vi "DriveModuleControl_TravTuneKsKv.vi"(8 "error in":errorcluster, 9 "Actual State":T1={"Speed"=0.0, "Angle"={"VALUE"=0.0, "COS"=1.0, "SIN"=0.0}} {"Angle"."SIN" format="%13.4f"; "Angle"."COS" format="%13.4f"; "Angle"."VALUE" format="%13.4f"}, 10 "Desired State":T1={"Speed"=0.0, "Angle"={"VALUE"=0.0, "COS"=1.0, "SIN"=0.0}} {"Angle"."SIN" format="%13.4f"; "Angle"."COS" format="%13.4f"; "Angle"."VALUE" format="%13.4f"}, 11 "ModualNamePrefix":i32) -> (0 "error out":errorcluster)   [LabVIEW 2023]
uses:
  <vilib>/Rock Robotics/WPI/ThirdParty/JAS_Junk/TrajLib/TypeDef/SWERVE_DRIVE_MODULE_STATE.ctl
  <vilib>/Rock Robotics/WPI/ThirdParty/JAS_Junk/TrajLib/TypeDef/ROTATION2D.ctl
  <vilib>/Rock Robotics/WPI/ThirdParty/JAS_Junk/TrajLib/Rotation2d_Minus.vi
  <vilib>/Rock Robotics/WPI/ThirdParty/JAS_Junk/TrajLib/Rotation2d_GetRadians.vi
  <vilib>/Rock Robotics/WPI/ThirdParty/JAS_Junk/TrajLib/SwerveModuleState_New.vi
  <vilib>/Rock Robotics/WPI/ThirdParty/JAS_Junk/TrajLib/Rotation2d_RotateBy.vi
  <vilib>/Rock Robotics/WPI/ThirdParty/JAS_Junk/TrajLib/Rotation2d_CreateAngle.vi
  <vilib>/Rock Robotics/WPI/ThirdParty/JAS_Junk/TrajLib/SimpleMotorFF_Calculate.vi
  <vilib>/Rock Robotics/WPI/ThirdParty/JAS_Junk/TrajLib/PIDController_AtSetpoint.vi
  <vilib>/Rock Robotics/WPI/ThirdParty/JAS_Junk/TrajLib/PIDController_SetPIDF.vi
  <vilib>/Rock Robotics/WPI/ThirdParty/JAS_Junk/TrajLib/PIDController_SetDerivativeFilter.vi
  <vilib>/Rock Robotics/WPI/ThirdParty/JAS_Junk/TrajLib/PIDController_SetIntegratorRange.vi
  <vilib>/Rock Robotics/WPI/ThirdParty/JAS_Junk/TrajLib/PIDController_SetTolerancePandV.vi
  <vilib>/Rock Robotics/WPI/ThirdParty/JAS_Junk/TrajLib/PIDController_DisableContinousInput.vi
  <vilib>/Rock Robotics/WPI/ThirdParty/JAS_Junk/TrajLib/PIDController_EnableContinousInput.vi
  <vilib>/Rock Robotics/WPI/ThirdParty/JAS_Junk/TrajLib/PIDController_Reset.vi
  <vilib>/Rock Robotics/WPI/ThirdParty/JAS_Junk/TrajLib/PIDController_New.vi
  <vilib>/Rock Robotics/WPI/ThirdParty/JAS_Junk/TrajLib/PIDController_SetOutputLimits.vi
  <vilib>/Rock Robotics/WPI/ThirdParty/JAS_Junk/TrajLib/VI/PIDController_SetIntegratorZone.vi
  <vilib>/Rock Robotics/WPI/ThirdParty/JAS_Junk/TrajLib/LinearFilter_ResetToValue.vi
  <vilib>/Rock Robotics/WPI/ThirdParty/JAS_Junk/TrajLib/LinearFilter_Calculate.vi
  <vilib>/Rock Robotics/WPI/ThirdParty/JAS_Junk/TrajLib/Rotation2d_UnaryMinus.vi
  <vilib>/Rock Robotics/WPI/ThirdParty/JAS_Junk/TrajLib/Rotation2d_CreateXY.vi
  <vilib>/Rock Robotics/WPI/ThirdParty/JAS_Junk/TrajLib/PIDController_NewPeriod.vi
  <vilib>/Rock Robotics/WPI/ThirdParty/JAS_Junk/TrajLib/Util_CalcDist.vi
  <vilib>/Rock Robotics/SystemInterfaces/NetworkCommunication/NetComm_UsageReport_report.vi
  DriveGlobal.vi
  <vilib>/Rock Robotics/WPI/ThirdParty/Phoenix-LabVIEW/CANCoder/CTRE_Phoenix_CANcoder_RefNumRegistryGet.vi
  <vilib>/Rock Robotics/WPI/MotorControl/WPI_MotorControlRefNum Registry Get.vi
  <vilib>/Rock Robotics/Network Tables/NT Write Number.vi
  <vilib>/Rock Robotics/WPI/ThirdParty/JAS_Junk/TrajLib/LinearFilter_MovingAverage.vi
  <vilib>/Rock Robotics/WPI/ThirdParty/JAS_Junk/TrajLib/LinearFilter_LowPassBW1.vi
  <vilib>/Rock Robotics/WPI/ThirdParty/JAS_Junk/TrajLib/LinearFilter_LowPassBW2.vi
  <vilib>/Rock Robotics/WPI/ThirdParty/JAS_Junk/TrajLib/LinearFilter_HighPassBW1.vi
  <vilib>/Rock Robotics/WPI/ThirdParty/JAS_Junk/TrajLib/LinearFilter_HighPassBW2.vi
  <vilib>/Utility/semaphor.llb/Obtain Semaphore Reference.vi
  <vilib>/Rock Robotics/WPI/ThirdParty/JAS_Junk/TrajLib/Timer_Reset.vi
  <vilib>/Rock Robotics/WPI/ThirdParty/JAS_Junk/TrajLib/Globals/Util_LibraryGlobals.vi
  <vilib>/Rock Robotics/WPI/ThirdParty/JAS_Junk/TrajLib/PIDController_AdvCalculate_FF_Sp_Pv.vi
  <vilib>/Rock Robotics/WPI/ThirdParty/JAS_Junk/TrajLib/Trajectory_Library.lvlib
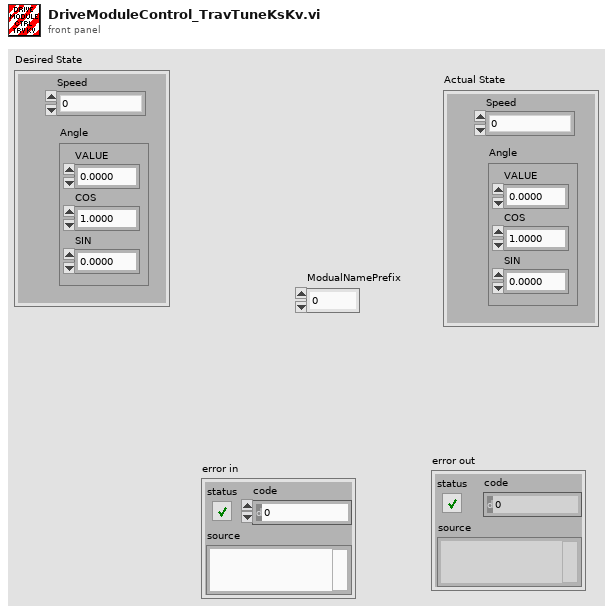
[diagram p1: front panel]
types:
  T1 = typedef "Trajectory_Library.lvlib/SWERVE_DRIVE_MODULE_STATE.ctl" = cluster{"Speed":dbl, "Angle":T2}
  T2 = typedef "Trajectory_Library.lvlib/ROTATION2D.ctl" = cluster{"VALUE":dbl, "COS":dbl, "SIN":dbl}
  T3 = enum16{"Moving Average", "Low Pass 1st Order Butterworth", "Low Pass 2nd Order Butterworth", "High Pass 1st Order Butterworth", "High Pass 2nd Order Butterworth"}
  T4 = typedef "WPI_MotorControlDeviceRef.ctl" = cluster{"DeviceStatus":errorcluster, "Type":T5, "PWM":cluster{"PWM Channel":T6, "DeadBand":T7}, "CAN":cluster{"Device Number":u8, "SetOutput VI Ref":variant, "GetOutput VI Ref":variant, "Enable VI Ref":variant, "Disable VI Ref":variant, "Data":variant}, "Invert":bool, "DIO PWM":cluster{"PWM \"Enable\" Channel":T6, "DIOChannel":T8, "PWM Rate":dbl}}
  T5 = typedef "WPI_MotorControlType.ctl" = enum16{"PWM", "CAN", "DIO PWM"}
  T6 = typedef "FPGA_DIOPWMChannel.ctl" = enum8{"PWM 0", "PWM 1", "PWM 2", "PWM 3", "PWM 4", "PWM 5", "PWM 6", "PWM 7", "PWM 8", "PWM 9", "PWM MXP 0", "PWM MXP 1", "PWM MXP 2", "PWM MXP 3", "PWM MXP 4", "PWM MXP 5", "PWM MXP 6", "PWM MXP 7", "PWM MXP 8", "PWM MXP 9", "Invalid"}
  T7 = typedef "WPI_PWMDeadband.ctl" = cluster{"Name":string, "maxPositivePwm":i32, "minPositivePwm":i32, "centerPwm":i32, "maxNegativePwm":i32, "minNegativePwm":i32, "angularRange":u16}
  T8 = typedef "FPGA_DIOChannel.ctl" = enum8{"DIO 0", "DIO 1", "DIO 2", "DIO 3", "DIO 4", "DIO 5", "DIO 6", "DIO 7", "DIO 8", "DIO 9", "DIO MXP 0", "DIO MXP 1", "DIO MXP 2", "DIO MXP 3", "DIO MXP 4", "DIO MXP 5", "DIO MXP 6", "DIO MXP 7", "DIO MXP 8", "DIO MXP 9", "DIO MXP 10", "DIO MXP 11", "DIO MXP 12", "DIO MXP 13", "DIO MXP 14", "DIO MXP 15", "SPI Port CS1", "SPI Port CS2", "SPI Port CS3", "SPI Port MISO", "SPI Port MOSI", "Invalid"}
  T9 = typedef "Trajectory_Library.lvlib/TIMER.ctl" = cluster{"StartTime":dbl, "Accumulated TIme":dbl, "Running":bool, "semaphore":T10}
  T10 = typedef "Semaphore RefNum" = refnum<k1>
  T11 = typedef "Trajectory_Library.lvlib/SIMPLE_MOTOR_FF.ctl" = cluster{"Ks":dbl, "Kv":dbl, "Ka":dbl, "KnInv":dbl}
  T12 = typedef "Trajectory_Library.lvlib/PID_ADV_LIMITS.ctl" = cluster{"MaxInput":dbl, "MinInput":dbl, "Continuous":bool, "MaxOutput":dbl, "MinOutput":dbl}
  T13 = typedef "Trajectory_Library.lvlib/PID_ADV_TUNING.ctl" = cluster{"Kf":dbl, "Kp":dbl, "Ki":dbl, "Kd":dbl, "MaximumIntegral":dbl, "MinimumIntegral":dbl, "Filter Derivative":bool, "IntegralZone":dbl}
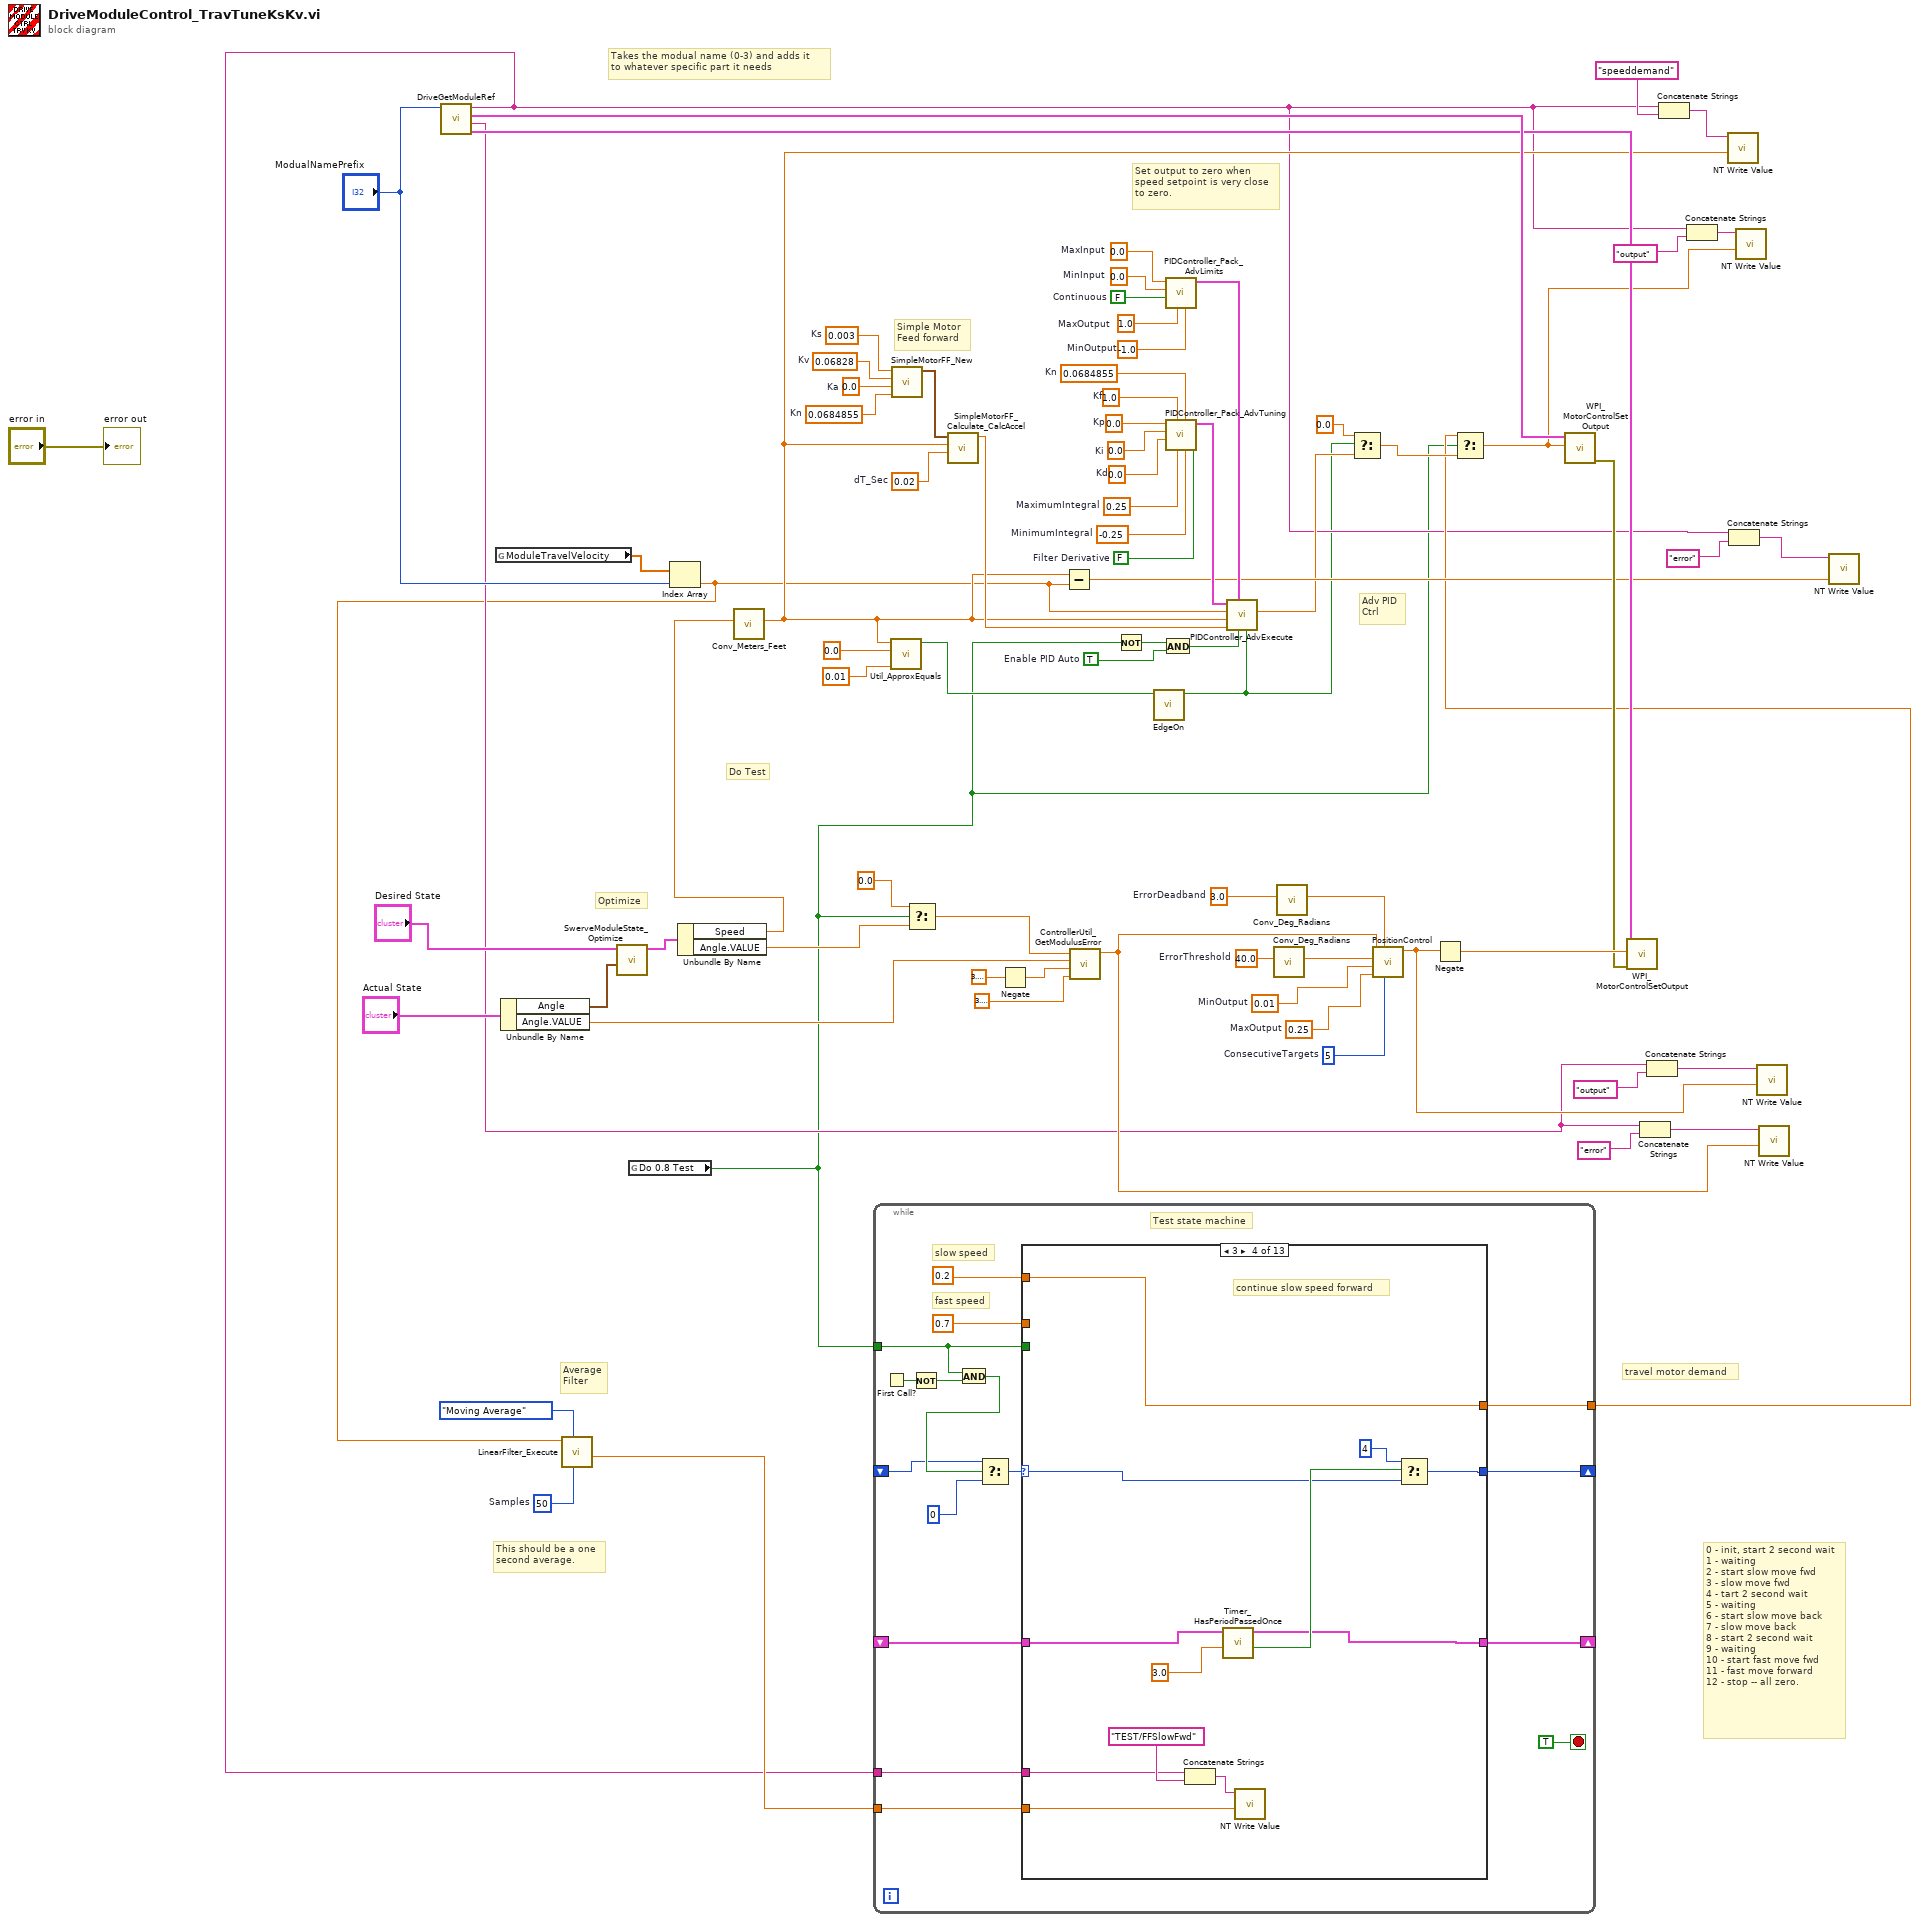
[diagram p0: block diagram]
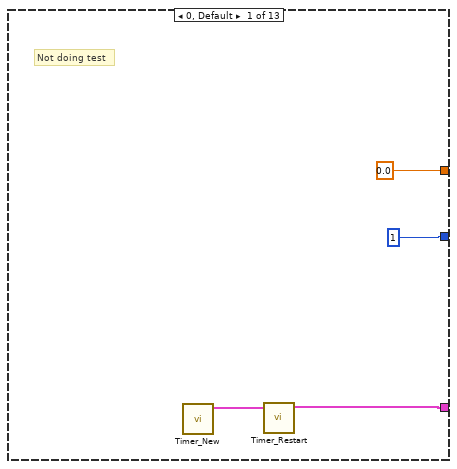
[diagram p2: hidden frame]
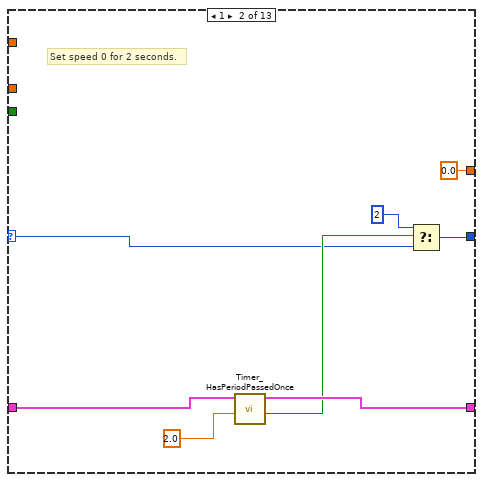
[diagram p3: hidden frame]
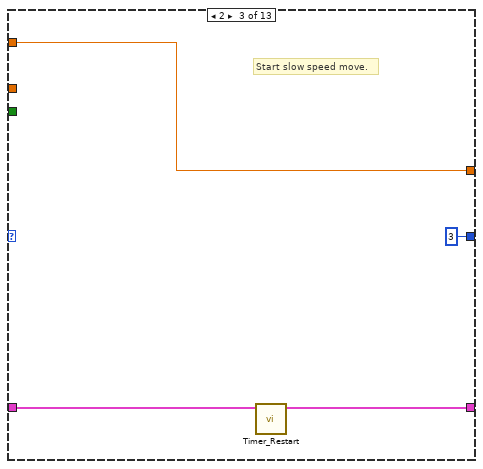
[diagram p4: hidden frame]
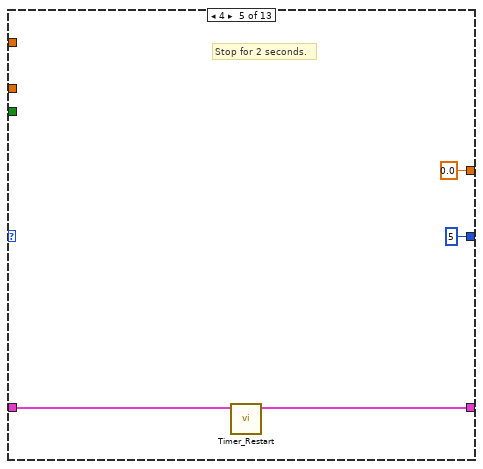
[diagram p5: hidden frame]
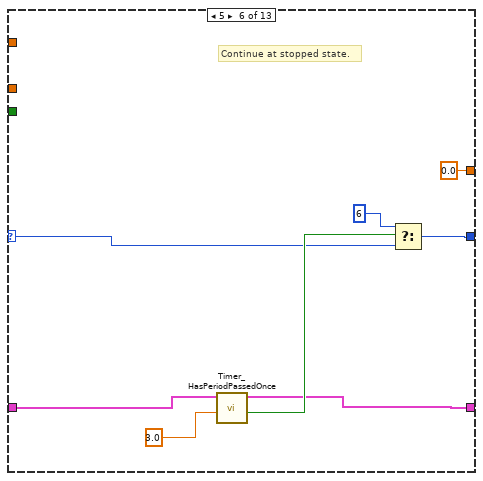
[diagram p6: hidden frame]
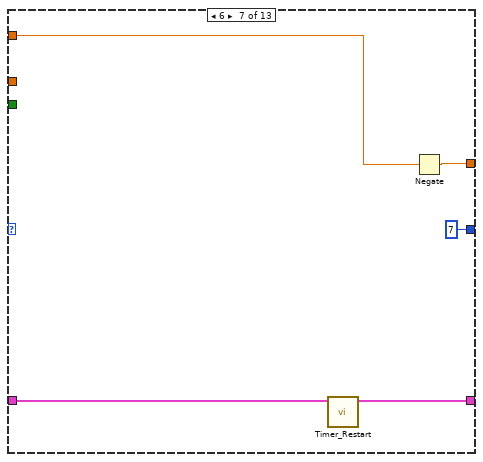
[diagram p7: hidden frame]
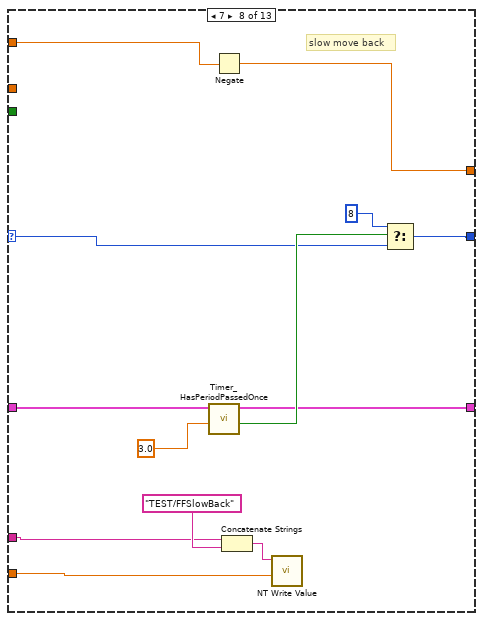
[diagram p8: hidden frame]
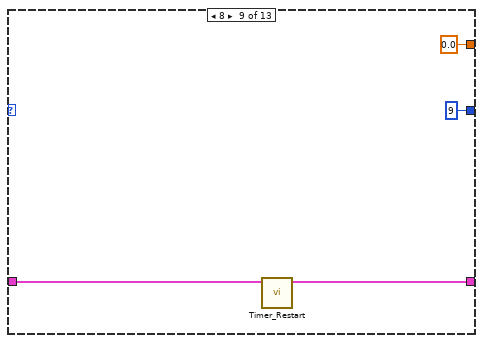
[diagram p9: hidden frame]
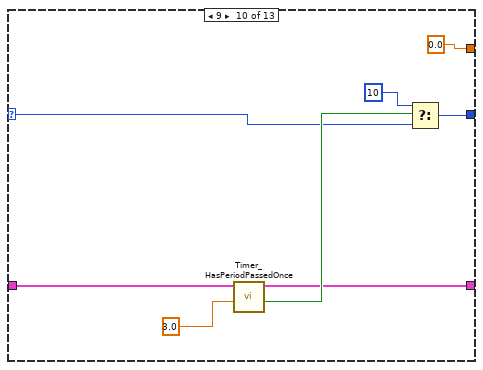
[diagram p10: hidden frame]
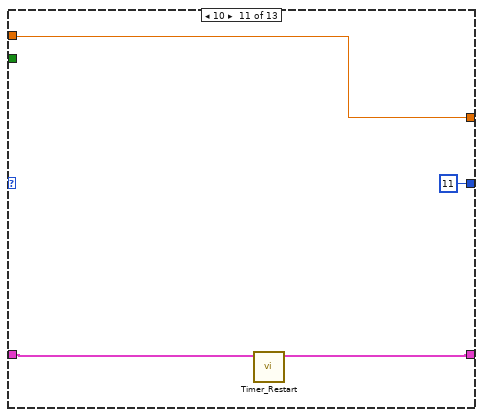
[diagram p11: hidden frame]
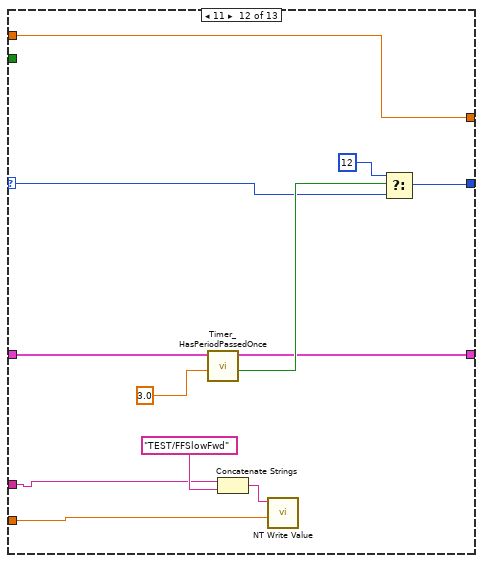
[diagram p12: hidden frame]
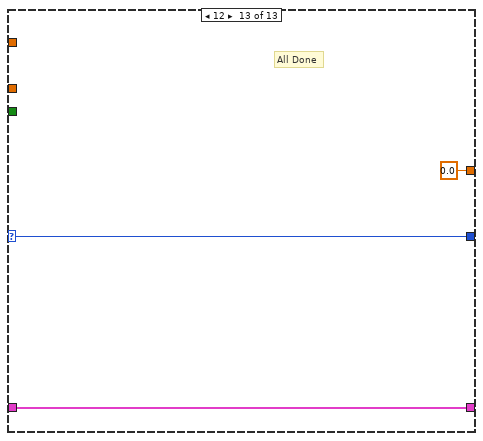
[diagram p13: hidden frame]
diagram:
  w8 = 50  # Samples
  w18 = TRUE  # Enable PID Auto
  w28 = 0.0684855  # Kn
  w45 = 0.0  # Kp
  w44 = 0.0  # Ki
  w43 = 0.0  # Kd
  w42 = 1.0  # Kf
  w41 = 0.25  # MaximumIntegral
  w40 = -0.25  # MinimumIntegral
  w39 = FALSE  # Filter Derivative
  w37 = 0.0  # MinInput
  w36 = FALSE  # Continuous
  w35 = 1.0  # MaxOutput
  w38 = -1.0  # MinOutput
  w34 = 0.0  # MaxInput
  w54 = 0.0684855  # Kn
  w53 = 0.02  # dT_Sec
  w51 = 0.003  # Ks
  w50 = 0.06828  # Kv
  w49 = 0.0  # Ka
  w64 = 5  # ConsecutiveTargets
  w61 = 0.25  # MaxOutput
  w65 = 0.01  # MinOutput
  w58 = 40.0  # ErrorThreshold
  w60 = 3.0  # ErrorDeadband
  # "This should be a one\nsecond average."
  # "Average\nFilter"
  # "0 - init, start 2 second wait\n1 - waiting\n2 - start slow move fwd\n3 - slow move fwd\n4 - tart 2 second wait\n5 - waiting\n6 - start slow move back\n7 - slow move back\n8 - start 2 second wait\n9 - waiting\n10 - start fast move fwd\n11 - fast move forward\n12 - stop -- all zero."
  # "travel motor demand"
  # "Do Test"
  # "Optimize"
  # "Set output to zero when\nspeed setpoint is very close\nto zero."
  # "Adv PID\nCtrl"
  # "Simple Motor\nFeed forward"
  # "Takes the modual name (0-3) and adds it \nto whatever specific part it needs"
  n1 = call "DriveGetModuleRef.vi"("ModualNamePrefix"="ModualNamePrefix") -> ("SpinMot"=w46:T4, "SpinStr"=w24:string, "TravMot"=w47:T4, "TravStr"=w4:string)  [unwired: 5 in, 2 out]
  n2 = global read "DriveGlobal.vi" "ModuleTravelVelocity"() -> (w30:dbl[])
  n3 = Unbundle By Name("Actual State") -> ("Angle"=w71:T2, "Angle.VALUE"=w68:dbl)
  n4 = call <vilib>:"SwerveModuleState_Optimize.vi"("CurrentAngle"=w71, "Desired State"="Desired State") -> ("out SWERVE_DRIVE_MODULE_STATE"=w69:T1)  [unwired: 9 in]
  n5 = global read "DriveGlobal.vi" "Do 0.8 Test"() -> (w1:bool)
  n6 = Index Array(array=w30, index="ModualNamePrefix") -> (element=w6:dbl)
  n7 = call <vilib>:"LinearFilter_Execute.vi"("Samples"=w8, "Filter Type"=T3."Moving Average", "Input"=w6) -> ("Output"=w5:dbl)  [unwired: 7 in, 1 out]
  n8 = Unbundle By Name(w69) -> ("Speed"=w15:dbl, "Angle.VALUE"=w14:dbl)
  n9 = call <vilib>:"Conv_Meters_Feet.vi"("Meters"=w15) -> ("Feet"=w21:dbl)  [unwired: 10 in]
  n10 = while {
    shift-right: [w96] -> _
    shift-left: _ -> [w88]
    shift-right: [w95] -> _
    shift-left: _ -> [w86]
    tunnel: w1 -> [w90]
    tunnel: [w87] -> w9
    tunnel: w5 -> [w83]
    tunnel: w4 -> [w82]
    stop <- TRUE stop-if-true
    # "fast speed"
    # "slow speed"
    # "Test state machine"
    n11 = First Call?() -> (First Call?: T/F=w92:bool)
    n12 = Not(x=w92) -> (.not. x?=w91:bool)
    n13 = And(x=w90, y=w91) -> (x .and. y?=w89:bool)
    n14 = Select(t=w88, s=w89, f=0 ("t")) -> (s? t:f=w94:i32)
    n15 = case shown="3" w94 {
      selector: w94 -> [_ w104 _ w121 _ w133 _ w149 _ w160 _ w176 w185]
      tunnel: [1 w103 3 ("t") w122 5 ("t") w134 7 ("t") w150 9 ("t") w164 11 ("t") w179 w185] -> w96
      tunnel: [w100 w107 w111 w119 w127 w131 w142 w147 w157 w162 w168 w177 w184] -> w95
      tunnel: w90 -> [_ _ _ _ _ _ _ _ _ _ _ _ _]
      tunnel: [0.0 0.0 w110 w118 0.0 0.0 w139 w154 0.0 0.0 w171 w183 0.0] -> w87
      tunnel: w86 -> [_ w108 w112 w120 w128 w132 w141 w148 w156 w163 w169 w178 w184]
      tunnel: 0.2 -> [_ _ w110 w118 _ _ w138 w155 _ _ _ _ _]
      tunnel: 0.7 -> [_ _ _ _ _ _ _ _ _ _ w171 w183 _]
      tunnel: w83 -> [_ _ _ w117 _ _ _ w143 _ _ _ w172 _]
      tunnel: w82 -> [_ _ _ w114 _ _ _ w144 _ _ _ w173 _]
      frame 0, Default {
        # "Not doing test"
        n16 = call <vilib>:"Timer_New.vi"() -> ("TIMER"=w101:T9)  [unwired: 11 in]
        n17 = call <vilib>:"Timer_Restart.vi"("in Timer"=w101) -> ("out Timer"=w100:T9)  [unwired: 10 in]
      }
      frame 1 {
        # "Set speed 0 for 2 seconds."
        n18 = call <vilib>:"Timer_HasPeriodPassedOnce.vi"("Period"=2.0, "in Timer"=w108) -> ("Expired"=w105:bool, "out Timer"=w107:T9)  [unwired: 7 in, 1 out]
        n19 = Select(t=2, s=w105, f=w104) -> (s? t:f=w103:i32)
      }
      frame 2 {
        # "Start slow speed move."
        n20 = call <vilib>:"Timer_Restart.vi"("in Timer"=w112) -> ("out Timer"=w111:T9)  [unwired: 10 in]
      }
      frame 3 {
        # "continue slow speed forward"
        n21 = Concatenate Strings(w114, "TEST/FFSlowFwd" ("refnum name")) -> (w115:string)
        n22 = call <vilib>:"Timer_HasPeriodPassedOnce.vi"("Period"=3.0, "in Timer"=w120) -> ("Expired"=w124:bool, "out Timer"=w119:T9)  [unwired: 7 in, 1 out]
        n23 = call-poly <vilib>:"NT Write Value.vi"("value"=w117, "name"=w115) -> ()  [unwired: 9 in, 1 out]
        n24 = Select(t=4, s=w124, f=w121) -> (s? t:f=w122:i32)
      }
      frame 4 {
        # "Stop for 2 seconds."
        n25 = call <vilib>:"Timer_Restart.vi"("in Timer"=w128) -> ("out Timer"=w127:T9)  [unwired: 10 in]
      }
      frame 5 {
        # "Continue at stopped state."
        n26 = call <vilib>:"Timer_HasPeriodPassedOnce.vi"("Period"=3.0, "in Timer"=w132) -> ("Expired"=w136:bool, "out Timer"=w131:T9)  [unwired: 7 in, 1 out]
        n27 = Select(t=6, s=w136, f=w133) -> (s? t:f=w134:i32)
      }
      frame 6 {
        n28 = call <vilib>:"Timer_Restart.vi"("in Timer"=w141) -> ("out Timer"=w142:T9)  [unwired: 10 in]
        n29 = Negate(x=w138) -> (-x=w139:dbl)
      }
      frame 7 {
        # "slow move back"
        n30 = call <vilib>:"Timer_HasPeriodPassedOnce.vi"("Period"=3.0, "in Timer"=w148) -> ("Expired"=w152:bool, "out Timer"=w147:T9)  [unwired: 7 in, 1 out]
        n31 = Negate(x=w155) -> (-x=w154:dbl)
        n32 = Concatenate Strings(w144, "TEST/FFSlowBack" ("refnum name")) -> (w145:string)
        n33 = call-poly <vilib>:"NT Write Value.vi"("value"=w143, "name"=w145) -> ()  [unwired: 9 in, 1 out]
        n34 = Select(t=8, s=w152, f=w149) -> (s? t:f=w150:i32)
      }
      frame 8 {
        n35 = call <vilib>:"Timer_Restart.vi"("in Timer"=w156) -> ("out Timer"=w157:T9)  [unwired: 10 in]
      }
      frame 9 {
        n36 = call <vilib>:"Timer_HasPeriodPassedOnce.vi"("Period"=3.0, "in Timer"=w163) -> ("Expired"=w166:bool, "out Timer"=w162:T9)  [unwired: 7 in, 1 out]
        n37 = Select(t=10, s=w166, f=w160) -> (s? t:f=w164:i32)
      }
      frame 10 {
        n38 = call <vilib>:"Timer_Restart.vi"("in Timer"=w169) -> ("out Timer"=w168:T9)  [unwired: 10 in]
      }
      frame 11 {
        n39 = call <vilib>:"Timer_HasPeriodPassedOnce.vi"("Period"=3.0, "in Timer"=w178) -> ("Expired"=w181:bool, "out Timer"=w177:T9)  [unwired: 7 in, 1 out]
        n40 = Concatenate Strings(w173, "TEST/FFSlowFwd" ("refnum name")) -> (w174:string)
        n41 = call-poly <vilib>:"NT Write Value.vi"("value"=w172, "name"=w174) -> ()  [unwired: 9 in, 1 out]
        n42 = Select(t=12, s=w181, f=w176) -> (s? t:f=w179:i32)
      }
      frame 12 {
        # "All Done"
      }
    }
  }
  n43 = call <vilib>:"Util_ApproxEquals.vi"("Tolerance"=0.01, "Value 2"=0.0, "Value 1"=w21) -> ("ApproxEquals"=w3:bool)  [unwired: 8 in]
  n44 = call <vilib>:"SimpleMotorFF_New.vi"("Kn"=w54, "Ka"=w49, "Kv"=w50, "Ks"=w51) -> ("SIMPLE_MOTOR_FF"=w52:T11)  [unwired: 7 in]
  n45 = Select(t=0.0, s=w1, f=w14) -> (s? t:f=w10:dbl)
  n46 = call <vilib>:"SimpleMotorFF_Calculate_CalcAccel.vi"("dT_Sec"=w53, "VelSp"=w21, "SIMPLE_MOTOR_FF"=w52) -> ("FeedForward"=w31:dbl)  [unwired: 8 in]
  n47 = Negate(x=3.141592653589793) -> (-x=w70:dbl)
  n48 = Subtract(x=w21, y=w6) -> (x-y=w25:dbl)
  n49 = call <vilib>:"ControllerUtil_GetModulusError.vi"("Maximum_Input"=3.141592653589793, "Minimum_Input"=w70, "Measurerment(PV)"=w68, "Reference(SP)"=w10) -> ("Error"=w62:dbl)  [unwired: 7 in]
  n50 = Not(x=w1) -> (.not. x?=w19:bool)
  n51 = call "EdgeOn.vi"("Current State"=w3) -> ("Edge On Found"=w2:bool)  [unwired: 10 in]
  n52 = And(x=w19, y=w18) -> (x .and. y?=w20:bool)
  n53 = call <vilib>:"PIDController_Pack_AdvLimits.vi"("MinOutput"=w38, "MaxOutput"=w35, "Continuous"=w36, "MinInput"=w37, "MaxInput"=w34) -> ("Adv PID Limits"=w32:T12)  [unwired: 6 in]
  n54 = call <vilib>:"PIDController_Pack_AdvTuning.vi"("Filter Derivative"=w39, "MinimumIntegral"=w40, "Kn"=w28, "MaximumIntegral"=w41, "Kf"=w42, "Kd"=w43, "Ki"=w44, "Kp"=w45) -> ("Adv PID Tuning"=w33:T13)  [unwired: 3 in]
  n55 = call <vilib>:"PIDController_AdvExecute.vi"("Reset"=w2, "Auto"=w20, "Adv PID Limits"=w32, "FF-FeedForward"=w31, "SP-SetPoint"=w21, "PV-Measurement"=w6, "Adv PID Tuning"=w33) -> ("CO-ControlOutput"=w17:dbl)  [unwired: 2 in, 2 out]
  n56 = call <vilib>:"Conv_Deg_Radians.vi"("Degress"=w58) -> ("Radians"=w57:dbl)  [unwired: 10 in]
  n57 = call <vilib>:"Conv_Deg_Radians.vi"("Degress"=w60) -> ("Radians"=w59:dbl)  [unwired: 10 in]
  n58 = Select(t=0.0, s=w2, f=w17) -> (s? t:f=w11:dbl)
  n59 = call "PositionControl.vi"("ConsecutiveTargets"=w64, "ErrorDeadband"=w59, "MaxOutput"=w61, "MinOutput"=w65, "ErrorThreshold"=w57, "Error"=w62) -> ("OutputValue"=w56:dbl)  [unwired: 3 in, 2 out]
  n60 = Negate(x=w56) -> (-x=w55:dbl)
  n61 = Select(t=w9, s=w1, f=w11) -> (s? t:f=w12:dbl)
  n62 = call <vilib>:"WPI_MotorControlSetOutput.vi"("Output"=w12, "MotorControlDevRef"=w47) -> ("error out"=w48:errorcluster)  [unwired: 7 in, 2 out]
  n63 = call <vilib>:"WPI_MotorControlSetOutput.vi"("error in (no error)"=w48, "Output"=w55, "MotorControlDevRef"=w46) -> ()  [unwired: 6 in, 3 out]
  n64 = Concatenate Strings(w24, "error" ("refnum name")) -> (w75:string)
  n65 = Concatenate Strings(w24, "output" ("refnum name")) -> (w63:string)
  n66 = Concatenate Strings(w4, "speeddemand" ("refnum name")) -> (w79:string)
  n67 = Concatenate Strings(w4, "output" ("refnum name")) -> (w77:string)
  n68 = call-poly <vilib>:"NT Write Value.vi"("value"=w21, "name"=w79) -> ()  [unwired: 9 in, 1 out]
  n69 = Concatenate Strings(w4, "error" ("refnum name")) -> (w26:string)
  n70 = call-poly <vilib>:"NT Write Value.vi"("value"=w12, "name"=w77) -> ()  [unwired: 9 in, 1 out]
  n71 = call-poly <vilib>:"NT Write Value.vi"("value"=w56, "name"=w63) -> ()  [unwired: 9 in, 1 out]
  n72 = call-poly <vilib>:"NT Write Value.vi"("value"=w62, "name"=w75) -> ()  [unwired: 9 in, 1 out]
  n73 = call-poly <vilib>:"NT Write Value.vi"("value"=w25, "name"=w26) -> ()  [unwired: 9 in, 1 out]
  "error out" <- "error in"
